vi "testDynamic Registration Example.vi"(8 "error in (no error)":errorcluster, 11 "TestCase in":refnum<class "Event Test Template Examples.lvclass">) -> (0 "error out":errorcluster, 3 "TestCase out":refnum<class "Event Test Template Examples.lvclass">)   [LabVIEW 2015, in "Event Test Template Examples.lvclass"]
uses:
  Event Test Template Examples.lvclass
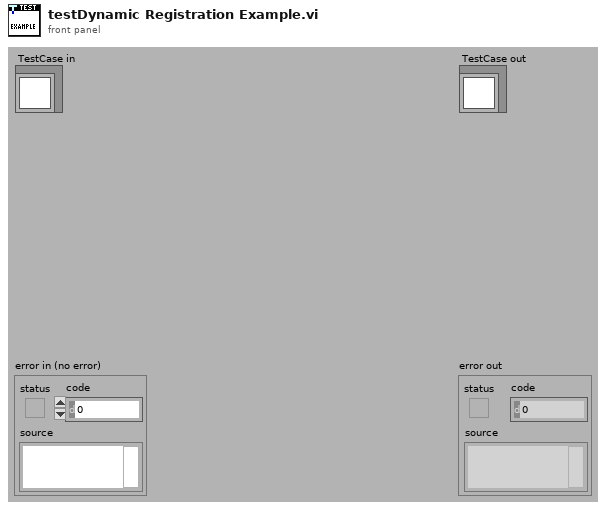
[diagram p1: front panel]
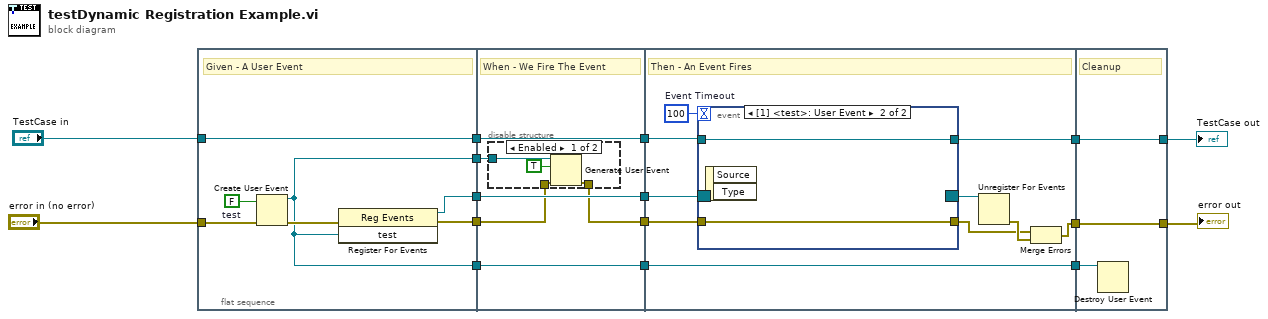
[diagram p0: block diagram]
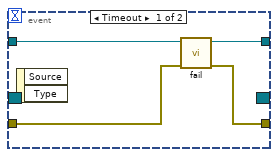
[diagram p3: hidden frame]
diagram:
  n1 = flat-sequence {
    tunnel: "error in (no error)" -> [w22]
    tunnel: "TestCase in" -> [w23]
    tunnel: [w23] -> w12
    tunnel: [w21] -> w11
    tunnel: [w18] -> w10
    tunnel: [w17] -> w9
    tunnel: [w17] -> w8
    tunnel: [w29] -> w7
    tunnel: w12 -> [w29]
    tunnel: [w28] -> w6
    tunnel: w11 -> [w28]
    tunnel: w10 -> [w27]
    tunnel: [w26] -> w5
    tunnel: w9 -> [w25]
    tunnel: w8 -> [w24]
    tunnel: [w24] -> w4
    tunnel: [w38] -> w3
    tunnel: [w37] -> w2
    tunnel: w7 -> [w39]
    tunnel: w6 -> [w40]
    tunnel: w5 -> [w36]
    tunnel: w4 -> [w35]
    tunnel: [w35] -> w1
    tunnel: [w52] -> w15
    tunnel: [w53] -> w13
    tunnel: w3 -> [w53]
    tunnel: w2 -> [w52]
    tunnel: w1 -> [w51]
    frame #0 {
      w19 = FALSE  # test
      # "Given - A User Event"
      n2 = Create User Event(user event datatype=w19, error in=w22) -> (user event=w17:refnum<user-event>, error out=w20:errorcluster)
      n3 = register-events(error in=w20, w17) -> (reference out=w21:refnum<event-registration>, error out=w18:errorcluster)  [unwired: 1 in]
    }
    frame #1 {
      # "When - We Fire The Event"
      n4 = disable-structure shown="Enabled" {
        disable-tunnel: w27 -> [w33 w34]
        disable-tunnel: [w32 w34] -> w26
        disable-tunnel: w25 -> [w31 _]
        frame Enabled {
          n5 = Generate User Event(user event=w31, event data cluster=TRUE ("event data"), error in=w33) -> (error out=w32:errorcluster)  [unwired: 1 in, 1 out]
        }
        frame Disabled {
        }
      }
    }
    frame #2 {
      w41 = 100  # Event Timeout
      # "Then - An Event Fires"
      n6 = event shown="[1] <test>: User Event" {
        selector: w40 -> [_ _]
        dyn-events: [_ _] -> w42
        timeout: w41 -> [_ _]
        tunnel: w39 -> [w48 w50]
        tunnel: [w47 w50] -> w38
        tunnel: [w46 w49] -> w43
        tunnel: w36 -> [w45 w49]
        event Timeout {
          n7 = event-data() -> ()  [unwired: 1 in, 2 out]
          n8 = call-dynamic "fail.vi"("error in (no error)"=w45, "TestCase in"=w48) -> ("error out"=w46:errorcluster, "TestCase out"=w47:refnum<class "Event Test Template Examples.lvclass">)  [unwired: 8 in]
        }
        event User Event {
          n9 = event-data() -> ()  [unwired: 1 in, 2 out]
        }
      }
      n10 = Unregister For Events(event registration refnum=w42) -> (error out=w44:errorcluster)  [unwired: 1 in]
      n11 = Merge Errors(w43, w44) -> (w37:errorcluster)
    }
    frame #3 {
      # "Cleanup"
      n12 = Destroy User Event(user event=w51) -> ()  [unwired: 1 in, 1 out]
    }
  }
  "error out" <- w15
  "TestCase out" <- w13
